vi "map_loading.vi"(3 "map file":path) -> (1 "status array":u8[][](array[numeric]))   [LabVIEW 2018]
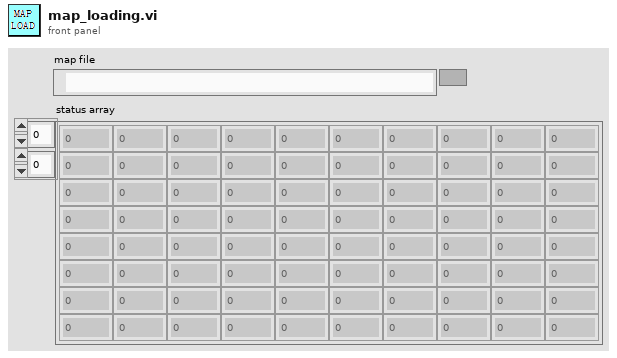
[diagram p1: front panel]
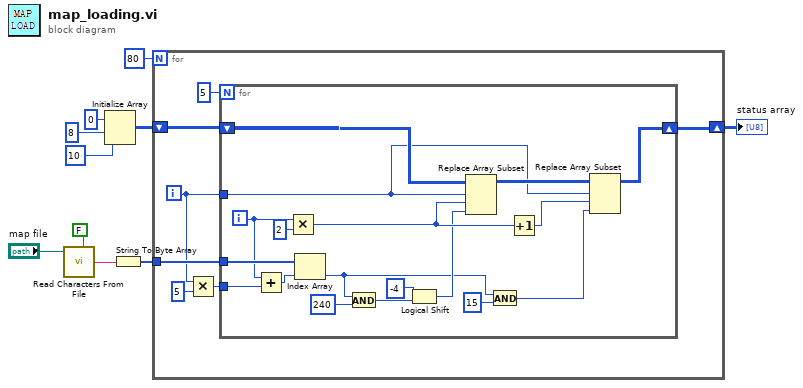
[diagram p0: block diagram]
diagram:
  n1 = call <vilib>:"Read Characters From File.vi"("file path (dialog if empty)"="map file", "convert eol? (no:F)"=FALSE) -> ("character string"=w9:string)  [unwired: 4 in, 3 out]
  n2 = Initialize Array(u8 0 ("element"), 8 ("dimension size"), 10 ("dimension size")) -> (w4:u8[][])
  n3 = String To Byte Array(string=w9) -> (unsigned byte array=w8:u8[])
  n4 = for {
    N: 80 -> [_]
    tunnel: w8 -> [w17]
    shift-right: [w14] -> w3
    shift-left: w4 -> [w16]
    i -> [w13]
    n5 = Multiply(x=w13, y=5) -> (x*y=w11:i32)
    n6 = for {
      N: 5 -> [_]
      tunnel: w17 -> [w25]
      shift-right: [w34] -> w14
      shift-left: w16 -> [w35]
      tunnel: w13 -> [w27]
      tunnel: w11 -> [w19]
      i -> [w20]
      n7 = Add(x=w20, y=w19) -> (x+y=w18:i32)
      n8 = Multiply(x=w20, y=2) -> (x*y=w29:i32)
      n9 = Index Array(array=w25, index=w18) -> (element=w21:u8)
      n10 = And(x=w21, y=u8 240) -> (x .and. y?=w24:u8)
      n11 = Logical Shift(y=i8 -4, x=w24) -> (x << y=w22:u8)
      n12 = Replace Array Subset(array=w35, new element=w22, index (row)=w27, index (col)=w29) -> (w33:u8[][])
      n13 = And(x=w21, y=u8 15) -> (x .and. y?=w26:u8)
      n14 = Increment(x=w29) -> (x+1=w28:i32)
      n15 = Replace Array Subset(array=w33, new element=w26, index (row)=w27, index (col)=w28) -> (w34:u8[][])
    }
  }
  "status array" <- w3
